vi "test Script APU.vi"(8 "error in (no error)":errorcluster, 11 "TestCase in":refnum<class "Scripting API Test Case.lvclass">) -> (0 "error out":errorcluster, 3 "TestCase out":refnum<class "Scripting API Test Case.lvclass">)   [LabVIEW 2015, in "Scripting API Test Case.lvclass"]
uses:
  Scripting API Test Case.lvclass
  SysDef API/Engine Simulation Toolkit Custom Device Settings.ctl
  <vilib>/NI Veristand/Custom Device API/Custom Device Timed Loop Priority.ctl
  SysDef API/APU Settings.ctl
  NationalInstruments.VeriStand.SystemDefinitionAPI
  <userlib>/_OpenG.lib/file/file.llb/Append Path to Root if Relative - Scalar__ogtk.vi
  <vilib>/addons/_JKI Toolkits/VI Tester/TestCase.llb/TestCase.lvclass
  SysDef API/Engine Simulation Toolkit SysDef API.lvlib
  <vilib>/NI VeriStand/Custom Device API/Custom Device API.lvlib
  niveristand-custom-device-testing-tools/VeriStandTestUtilities/VeriStandTestUtilities.lvlib
panel:
  out "string":string
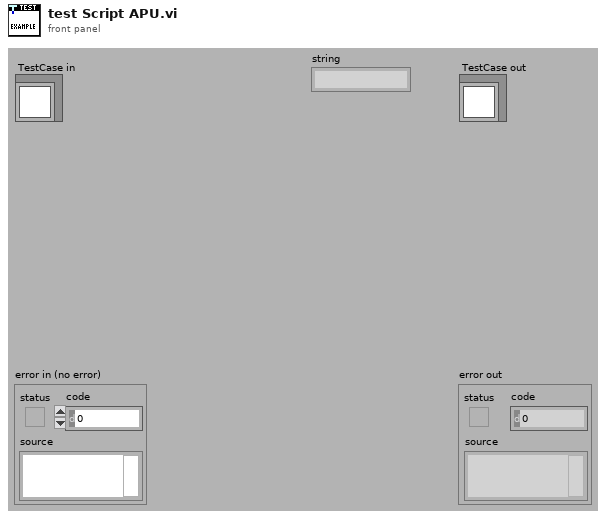
[diagram p1: front panel]
types:
  T1 = typedef "Engine Simulation Toolkit SysDef API.lvlib/Engine Simulation Toolkit Custom Device Settings.ctl" = cluster{"Name":string, "Execution priority":T2, "Rate decimation":i32, "CPU":i32, "Device address":string, "Bitfile path":path}
  T2 = typedef "Custom Device API.lvlib/Custom Device Timed Loop Priority.ctl" = enum32{"Low", "Medium", "High"}
  T3 = typedef "Engine Simulation Toolkit SysDef API.lvlib/APU Settings.ctl" = cluster{"Start angle (degrees)":dbl, "Start speed (RPM)":dbl, "Engine accelerates to RPM set points":bool, "Acceleration (RPM/sec)":dbl}
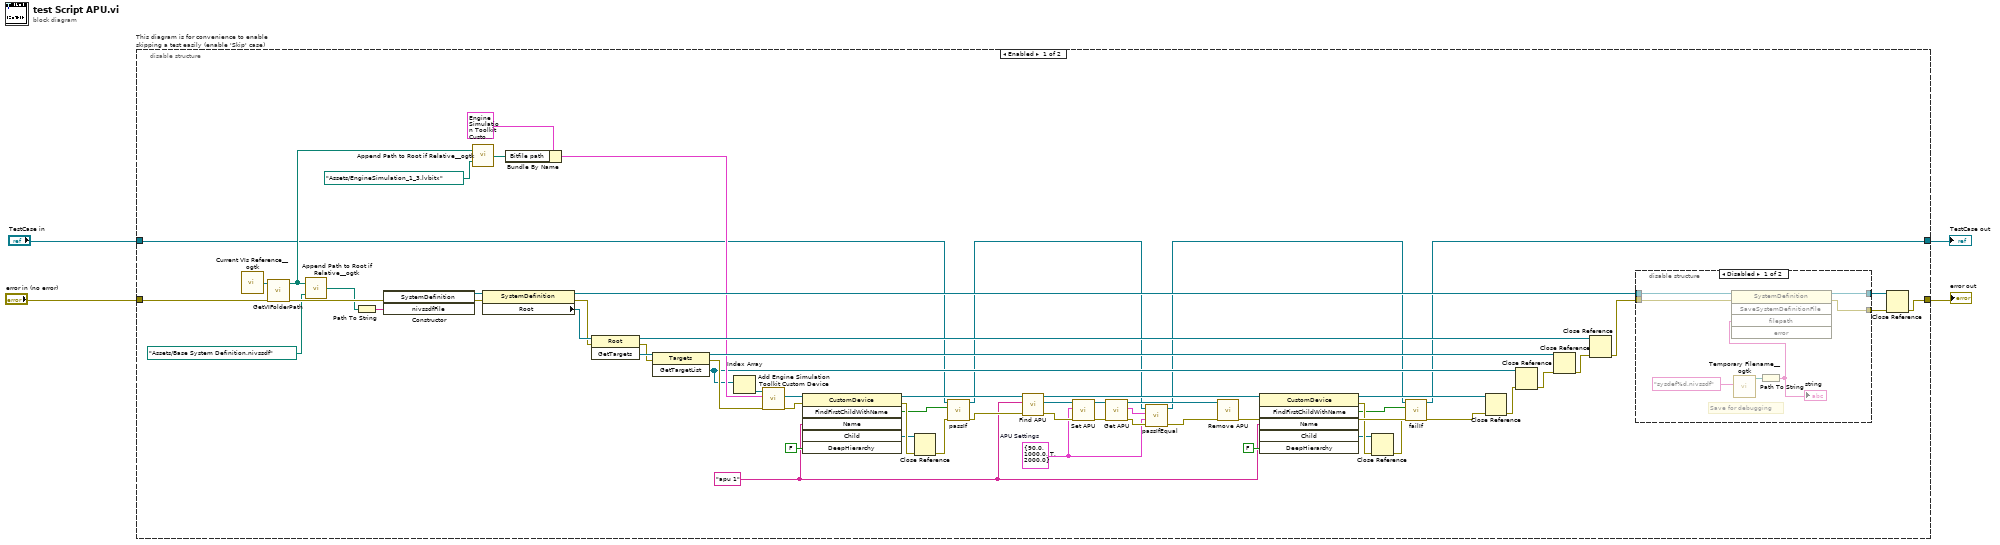
[diagram p0: block diagram]
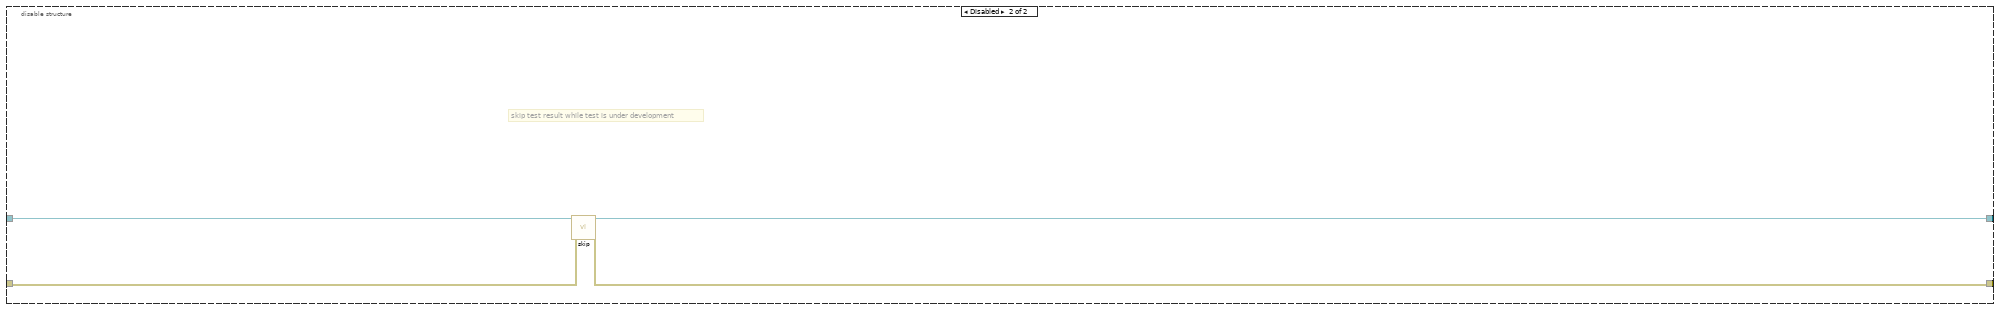
[diagram p3: hidden frame]
diagram:
  n1 = disable-structure "This diagram is for convenience to enable skipping a test easily (enable 'Skip' case)" shown="Enabled" {
    disable-tunnel: "TestCase in" -> [w16 w78]
    disable-tunnel: [w17 w76] -> w1
    disable-tunnel: [w57 w77] -> w3
    disable-tunnel: "error in (no error)" -> [w43 w75]
    frame Enabled {
      w5 = T3 {"Start angle (degrees)"=90.0, "Start speed (RPM)"=1000.0, "Engine accelerates to RPM set points"=TRUE, "Acceleration (RPM/sec)"=2000.0}  # APU Settings
      w18 = "apu 1" ("APU name")
      n2 = call <userlib>:"Current VIs Reference__ogtk.vi"() -> ("Current VI's reference"=w44:refnum<vi>)  [unwired: 5 in]
      n3 = call "GetVIFolderPath.vi"("error in (no error)"=w43, "VI Reference in"=w44) -> ("error out"=w42:errorcluster, "VI Folder Path out"=w41:path)  [unwired: 8 in]
      n4 = call-poly <userlib>:"Append Path to Root if Relative__ogtk.vi"("Absolute or Relative Path"=path "Assets/Base System Definition.nivssdf", "Root Path"=w41) -> ("Absolute or Appended Path"=w37:path)
      n5 = Path To String(path=w37) -> (string=w45:string)
      n6 = constructor class="SystemDefinition"(error in=w42, "nivssdfFile"=w45) -> (reference out=w65:refnum<k24>, error out=w64:errorcluster)  [unwired: 2 in, 2 out]
      n7 = call-poly <userlib>:"Append Path to Root if Relative__ogtk.vi"("Absolute or Relative Path"=path "Assets/EngineSimulation_1_3.lvbitx", "Root Path"=w41) -> ("Absolute or Appended Path"=w46:path)
      n8 = property class="SystemDefinition"(reference=w65, error in=w64) -> (reference out=w58:refnum<k24>, error out=w60:errorcluster, "Root"=w63:refnum<k24>)
      n9 = Bundle By Name(cluster=T1 {"Name"="Engine Simulation Toolkit", "Execution priority"=enum."Medium", "Rate decimation"=1, "CPU"=-2, "Device address"="RIO 0", "Bitfile path"=path ""} ("Engine Simulation Toolkit Custom Device Settings"), "Bitfile path"=w46) -> (w48:T1)
      n10 = invoke class="Root" method="GetTargets"(reference=w63, error in=w60) -> (reference out=w53:refnum<k24>, error out=w61:errorcluster, "GetTargets"=w62:refnum<k24>)  [unwired: 1 in]
      n11 = invoke class="Targets" method="GetTargetList"(reference=w62, error in=w61) -> (reference out=w52:refnum<k24>, error out=w49:errorcluster, "GetTargetList"=w39:refnum<k24>[])  [unwired: 1 in]
      n12 = Index Array(array=w39) -> (element=w40:refnum<k24>)  [unwired: 1 in]
      n13 = call "Add Engine Simulation Toolkit Custom Device.vi"("error in (no error)"=w49, "Engine Simulation Toolkit Custom Device Settings"=w48, "Target in"=w40) -> ("error out"=w34:errorcluster, "EST Custom Device"=w27:refnum<k24>)  [unwired: 6 in, 1 out]
      n14 = invoke class="CustomDevice" method="FindFirstChildWithName"(reference=w27, error in=w34, "Name"=w18, "DeepHierarchy"=FALSE) -> (reference out=w26:refnum<k24>, error out=w30:errorcluster, "FindFirstChildWithName"=w28:bool, "Child"=w29:refnum<k24>)  [unwired: 2 in, 2 out]
      n15 = Close Reference(reference=w29, error in (no error)=w30) -> (error out=w31:errorcluster)
      n16 = call-dynamic "passIf.vi"("error in (no error)"=w31, "pass"=w28, "TestCase in"=w16) -> ("error out"=w33:errorcluster, "TestCase out"=w8:refnum<class "Scripting API Test Case.lvclass">)  [unwired: 7 in]
      n17 = call "Find APU.vi"("error in (no error)"=w33, "APU name"=w18, "EST custom device in"=w26) -> ("error out"=w14:errorcluster, "APU Node"=w15:refnum<k24>, "EST custom device out"=w20:refnum<k24>)  [unwired: 6 in]
      n18 = call "Set APU.vi"("error in (no error)"=w14, "APU Settings"=w5, "APU Node"=w15) -> ("error out"=w12:errorcluster, "APU Node"=w13:refnum<k24>)  [unwired: 7 in]
      n19 = call "Get APU.vi"("error in (no error)"=w12, "APU Node"=w13) -> ("error out"=w9:errorcluster, "APU Settings"=w6:T3, "APU Node"=w11:refnum<k24>)  [unwired: 7 in]
      n20 = call-dynamic "passIfEqual.vi"("error in (no error)"=w9, "y"=w5, "x"=w6, "TestCase in"=w8) -> ("error out"=w10:errorcluster, "TestCase out"=w7:refnum<class "Scripting API Test Case.lvclass">)  [unwired: 6 in]
      n21 = call "Remove APU.vi"("error in (no error)"=w10, "APU Node"=w11) -> ("error out"=w35:errorcluster)  [unwired: 9 in]
      n22 = invoke class="CustomDevice" method="FindFirstChildWithName"(reference=w20, "Name"=w18, "DeepHierarchy"=FALSE) -> (reference out=w19:refnum<k24>, error out=w23:errorcluster, "FindFirstChildWithName"=w21:bool, "Child"=w22:refnum<k24>)  [unwired: 3 in, 2 out]
      n23 = Close Reference(reference=w22, error in (no error)=w23) -> (error out=w24:errorcluster)
      n24 = call-dynamic "failIf.vi"("error in (no error)"=w24, "fail"=w21, "TestCase in"=w7) -> ("TestCase out"=w17:refnum<class "Scripting API Test Case.lvclass">)  [unwired: 7 in, 1 out]
      n25 = Close Reference(reference=w19, error in (no error)=w35) -> (error out=w36:errorcluster)
      n26 = Close Reference(reference=w39, error in (no error)=w36) -> (error out=w50:errorcluster)
      n27 = Close Reference(reference=w52, error in (no error)=w50) -> (error out=w51:errorcluster)
      n28 = Close Reference(reference=w53, error in (no error)=w51) -> (error out=w54:errorcluster)
      n29 = disable-structure shown="Disabled" {
        disable-tunnel: w58 -> [w72 w73]
        disable-tunnel: [w71 w74] -> w56
        disable-tunnel: [w70 w73] -> w55
        disable-tunnel: w54 -> [w69 w74]
        frame Disabled {
          # "Save for debugging"
          n30 = call <userlib>:"Temporary Filename__ogtk.vi"("pattern (lvtemp%d.tmp)"="sysdef%d.nivssdf") -> ("file in tmp dir"=w67:path)  [unwired: 5 in, 1 out]
          n31 = Path To String(path=w67) -> (string=w66:string)
          "string" <- w66
          n32 = invoke class="SystemDefinition" method="SaveSystemDefinitionFile"(reference=w72, error in=w69, "filepath"=w66) -> (reference out=w70:refnum<k24>, error out=w71:errorcluster)  [unwired: 2 in, 3 out]
        }
        frame Enabled {
        }
      }
      n33 = Close Reference(reference=w55, error in (no error)=w56) -> (error out=w57:errorcluster)
    }
    frame Disabled {
      # "skip test result while test is under development"
      n34 = call <vilib>:"skip.vi"("error in (no error)"=w75, "TestCase in"=w78) -> ("error out"=w77:errorcluster, "TestCase out"=w76:refnum<class "Scripting API Test Case.lvclass">)  [unwired: 8 in]
    }
  }
  "error out" <- w3
  "TestCase out" <- w1
